vi "UHR-Fleezers Control (host) - 12.6.vi"() -> ()   [LabVIEW 2012] (continued)
          tunnel: w2733 -> [w2738]
          tunnel: [w2736] -> w2731
          tunnel: [w2735] -> w2730
          tunnel: [w2741] -> w2729
          tunnel: w2731 -> [w2741]
          tunnel: [w2740] -> w2728
          tunnel: w2730 -> [w2740]
          tunnel: w2729 -> [w2745]
          tunnel: w2728 -> [w2744]
          tunnel: [w2743] -> w2732
          frame #0 {
            n1852 = xnode "Read/Write Control"("FPGA VI Reference In"=w2739, "error in"=w2738, "Green Filter Flipper"=TRUE) -> ("FPGA VI Reference Out"=w2736:T20, "error out"=w2735:errorcluster)
          }
          frame #1 {
            n1853 = Wait (ms)(milliseconds to wait=u32 100) -> ()  [unwired: 1 out]
          }
          frame #2 {
            n1854 = xnode "Read/Write Control"("FPGA VI Reference In"=w2745, "error in"=w2744, "Green Filter Flipper"=FALSE) -> ("error out"=w2743:errorcluster)  [unwired: 1 out]
          }
        }
      }
      event "Pump 1 contents", "Pump 3 contents": Value Change {
        n1855 = event-data() -> ()  [unwired: 7 out]
        n1856 = local read "Pump 1 contents"() -> (→"Pump 1 cont disp":string)
        n1857 = local read "Pump 3 contents"() -> (→"Pump 3 cont disp":string)
      }
      event "Reset Trap Pos. FB": Value Change {
        n1858 = event-data() -> ()  [unwired: 7 out]
        n1859 = xnode "Read/Write Control"("FPGA VI Reference In"=w2751, "error in"=w2750, "Trap Pos. FB Reset"="Reset Trap Pos. FB") -> ()  [unwired: 2 out]
      }
      event "Rem fb disp offset": Value Change {
        n1860 = event-data() -> ()  [unwired: 7 out]
        n1861 = local write "Rem fb disp offset"(FALSE ("Rem fb disp offset")) -> ()
        n1862 = local read "Mean T1 Position (nm)"() -> (w2753:dbl)
        n1863 = local read "FB Trap Pos Offset"() -> (w2754:dbl)
        n1864 = Subtract(x=w2754, y=w2753) -> (x-y=w2752:dbl)
        n1865 = local write "FB Trap Pos Offset"(w2752) -> ()
      }
      event "Threshold (nm)": Value Change {
        n1866 = event-data() -> ()  [unwired: 7 out]
        n1867 = flat-sequence {
          tunnel: w2758 -> [w2766]
          tunnel: w2757 -> [w2765]
          tunnel: [w2759] -> w2756
          tunnel: w2756 -> [w2772]
          frame #0 {
            n1868 = xnode "Read/Write Control"("FPGA VI Reference In"=w2766, "error in"=w2765) -> ("FPGA VI Reference Out"=w2762:T20, "error out"=w2761:errorcluster, "FPGA TTrig Thresh"=w2763:i64)
            n1869 = local read "Threshold stored (nm)"() -> (w2771:dbl)
            n1870 = local read "Threshold (nm)"() -> (w2759:dbl)
            n1871 = local read "AOM X Cal (nm/MHz)"() -> (w2769:dbl)
            n1872 = Subtract(x=w2759, y=w2771) -> (x-y=w2770:dbl)
            n1873 = Divide(x=w2770, y=w2769) -> (x/y=w2767:dbl)
            n1874 = call "IR AOM freq to word.vi"("Frequency In (MHz)"=w2767) -> ("Frequency Word Out (double)"=w2768:dbl)
            n1875 = To Quad Integer(1:w2768) -> (0:w2764:i64)
            n1876 = Add(x=w2763, y=w2764) -> (x+y=w2760:i64)
            n1877 = xnode "Read/Write Control"("FPGA VI Reference In"=w2762, "error in"=w2761, "FPGA TTrig Thresh"=w2760) -> ()  [unwired: 2 out]
          }
          frame #1 {
            "Threshold stored (nm)" <- w2772
          }
        }
      }
      event "FB Trig Integrate": Value Change {
        n1878 = event-data() -> ()  [unwired: 7 out]
        n1879 = local read "FB Trig Integrate"() -> (w2774:u32)
        n1880 = xnode "Read/Write Control"("FPGA VI Reference In"=w2776, "error in"=w2775, "FB Trig Integrate"=w2774) -> ("error out"=w2773:errorcluster)  [unwired: 1 out]
      }
      event "11": Value Change {
        n1881 = event-data() -> ()  [unwired: 7 out]
        n1882 = local read "11"() -> (w2777:bool)
        n1883 = case shown="True" w2777 {
          frame False {
          }
          frame True {
            n1884 = local read "Messages"() -> (w2779:string)
            n1885 = call "Update messages.vi"("Message to add"="You kicked it up to 11!", "Old message string"=w2779) -> ("New message string"=w2780:string)
            n1886 = call <vilib>:"Beep.vi"() -> ()  [unwired: 12 in]
            n1887 = local write "Messages"(w2780) -> ()
          }
        }
      }
      event "Trap Pos. FB ON": Value Change {
        n1888 = event-data() -> ()  [unwired: 7 out]
        n1889 = xnode "Read/Write Control"("FPGA VI Reference In"=w2783, "error in"=w2782, "Force feedback"="Trap Pos. FB ON") -> ()  [unwired: 2 out]
      }
      event "Remove Action Offset": Value Change {
        n1890 = event-data() -> ()  [unwired: 7 out]
        n1891 = local write "Remove Action Offset"(FALSE ("Remove Action Offset")) -> ()
        n1892 = local read "Trap Pos. FB Mult Factor"() -> (w2788:i64)
        n1893 = local read "Trap Pos FB Action"() -> (w2786:i64)
        n1894 = local read "Trap Pos. FB Offset Factor"() -> (w2784:i64)
        n1895 = Multiply(x=w2788, y=w2786) -> (x*y=w2787:i64)
        n1896 = Add(x=w2787, y=w2784) -> (x+y=w2785:i64)
        n1897 = local write "Trap Pos. FB Offset Factor"(w2785) -> ()
        n1898 = xnode "Read/Write Control"("FPGA VI Reference In"=w2791, "error in"=w2790, "Trap Pos. FB Offset Factor"=w2785) -> ()  [unwired: 2 out]
      }
      event "Remove Unwinding Offset": Value Change {
        n1899 = event-data() -> ()  [unwired: 7 out]
        n1900 = local write "Remove Unwinding Offset"(FALSE ("Remove Action Offset")) -> ()
        n1901 = local read "Trap Pos. FB Mult Factor"() -> (w2803:i64)
        n1902 = local read "Trap Pos FB Action"() -> (w2801:i64)
        n1903 = local read "Trap Pos. FB Offset Factor"() -> (w2800:i64)
        n1904 = Multiply(x=w2803, y=w2801) -> (x*y=w2802:i64)
        n1905 = local read "Trap Pos. FB Mult Factor"() -> (w2799:i64)
        n1906 = Add(x=w2802, y=w2800) -> (x+y=w2793:i64)
        n1907 = Multiply(x=32768, y="factor") -> (x*y=w2796:dbl)
        n1908 = Multiply(x=w2796, y=w2799) -> (x*y=w2798:dbl)
        n1909 = Subtract(x=w2793, y=w2798) -> (x-y=w2797:dbl)
        n1910 = To Quad Integer(1:w2797) -> (0:w2792:i64)
        n1911 = xnode "Read/Write Control"("FPGA VI Reference In"=w2806, "error in"=w2805, "Trap Pos. FB Offset Factor"=w2792) -> ()  [unwired: 2 out]
        n1912 = local write "Trap Pos. FB Offset Factor"(w2792) -> ()
      }
      event "Trap Pos. FB Range", "Trap Pos. FB Gains", "Trap Pos. FB Mult Factor", "Trap Pos. FB Offset Factor", "Trap Pos FB Negate Action", "Trap Pos FB Monitor\nT1 or T2", "Differential FB?", "Negate Diff?": Value Change {
        n1913 = event-data() -> ()  [unwired: 7 out]
        n1914 = Unbundle By Name("Trap Pos. FB Gains") -> ("proportional gain (Kc)"=w2809:fxp<+/-,16,8>, "integral gain (Kc*Ts/Ti)"=w2808:fxp<+/-,16,8>, "derivative gain (Kc*Td/Ts)"=w2807:fxp<+/-,16,8>)
        n1915 = local read "Negate Diff?"() -> (w2814:bool)
        n1916 = Unbundle By Name("Trap Pos. FB Range") -> ("output high"=w2812:fxp<+/-,16,1>, "output low"=w2811:fxp<+/-,16,1>)
        n1917 = xnode "Read/Write Control"("FPGA VI Reference In"=w2822, "error in"=w2821, "FB2 output high"=w2812, "FB2 output low"=w2811, "P2"=w2809, "I2"=w2808, "D2"=w2807, "Trap Pos. FB Mult Factor"="Trap Pos. FB Mult Factor", "Trap Pos. FB Offset Factor"="Trap Pos. FB Offset Factor", "Trap Pos FB Negate Action"="Trap Pos FB Negate Action", "Trap Pos FB Monitor T1 or T2"="Trap Pos FB Monitor\nT1 or T2", "AI1 X Scale"="Trap Pos. AI1 X Pre-scale", "Negate Diff?"=w2814, "Diff FB Measurement?"="Differential FB?") -> ()  [unwired: 2 out]
      }
      event "Trap Pos FB SP", "Trap Pos FB SP 2", "Use SP 2": Value Change {
        n1918 = event-data() -> ()  [unwired: 7 out]
        n1919 = Select(t="Trap Pos FB SP 2", s="Use SP 2", f="Trap Pos FB SP") -> (s? t:f=w2823:fxp<+/-,16,1>)
        n1920 = xnode "Read/Write Control"("FPGA VI Reference In"=w2828, "error in"=w2827, "Trap Pos. FB SP"=w2823) -> ()  [unwired: 2 out]
      }
      event "Offset SP2 from SP1": Value Change {
        n1921 = event-data() -> ()  [unwired: 7 out]
        n1922 = local read "Trap Pos FB SP"() -> (w2831:fxp<+/-,16,1>)
        n1923 = Add(x=w2831, y="SP2 Offset") -> (x+y=w2829:fxp<+/-,16,1>)
        n1924 = property on="Trap Pos FB SP 2" class="DigNum (strict)"("Val(Sgnl)"=w2829) -> ()  [unwired: 2 in, 2 out]
        n1925 = local write "Offset SP2 from SP1"(FALSE ("Offset SP2 from SP1")) -> ()
      }
      event "Set Reading to\nSetpoint": Value Change {
        # "This is the actual PID input signal"
        n1926 = event-data() -> ()  [unwired: 7 out]
        n1927 = local write "Set Reading to\nSetpoint"(FALSE ("Set SP to Reading")) -> ()
        n1928 = xnode "Read/Write Control"("FPGA VI Reference In"=w2837, "error in"=w2836) -> ("FPGA VI Reference Out"=w2835:T20, "error out"=w2834:errorcluster, "Trap Pos FB Int-Norm Signal"=w2833:fxp<+/-,16,1>)
        n1929 = local read "Differential FB?"() -> (w2838:bool)
        n1930 = case shown="False" w2838 {
          tunnel: [w2843 w2850] -> w2840
          tunnel: w2833 -> [w2841 w2850]
          frame False {
            n1931 = local read "Trap Pos FB Monitor\nT1 or T2"() -> (w2846:bool)
            n1932 = local read "Trap X AI1 (DMA)"() -> (w2849:T13)
            n1933 = Unbundle By Name(w2849) -> ("Set 1"=w2848:fxp<+/-,16,1>, "Set 2"=w2847:fxp<+/-,16,1>)
            n1934 = Select(t=w2848, s=w2846, f=w2847) -> (s? t:f=w2845:fxp<+/-,16,1>)
            n1935 = Not(x="Set SP Using...") -> (.not. x?=w2842:bool)
            n1936 = Select(t=w2841, s=w2842, f=w2845) -> (s? t:f=w2843:fxp<+/-,16,1>)
          }
          frame True {
          }
        }
        n1937 = xnode "Read/Write Control"("FPGA VI Reference In"=w2835, "error in"=w2834, "Trap Pos. FB SP"=w2840) -> ()  [unwired: 2 out]
        n1938 = local write "Trap Pos FB SP"(w2840) -> ()
      }
      event "Trap Pos. FB Out Scale 2^n": Value Change {
        n1939 = event-data() -> ()  [unwired: 7 out]
        n1940 = Scale By Power Of 2(n="Trap Pos. FB Out Scale 2^n", x=ext 1.0) -> (x*2^n=w2851:ext)
        n1941 = property on="Trap Pos. FB Mult Factor" class="DigNum (strict)"("Val(Sgnl)"=w2851) -> ()  [unwired: 2 in, 2 out]
      }
      event "Trap Pos FB Int Count": Value Change {
        n1942 = event-data() -> ()  [unwired: 7 out]
        n1943 = xnode "Read/Write Control"("FPGA VI Reference In"=w2856, "error in"=w2855, "Trap Pos FB Int Count"="Trap Pos FB Int Count") -> ()  [unwired: 2 out]
      }
      event "Trap pos": Value Change {
        n1944 = event-data() -> ()  [unwired: 7 out]
        n1945 = case shown="True" "Trap pos" {
          frame False {
            n1946 = property on="Trap Delta Graph" class="WFGraph (strict)"("Visible"=TRUE) -> ()  [unwired: 2 in, 2 out]
            n1947 = property on="Saved trap pos" class="WFGraph (strict)"("Visible"=FALSE) -> ()  [unwired: 2 in, 2 out]
          }
          frame True {
            n1948 = property on="Saved trap pos" class="WFGraph (strict)"("Visible"=TRUE) -> ()  [unwired: 2 in, 2 out]
            n1949 = property on="Trap Delta Graph" class="WFGraph (strict)"("Visible"=FALSE) -> ()  [unwired: 2 in, 2 out]
          }
        }
      }
    }
    "error out 2" <- w1685
    n1950 = node-c288() -> ()  [unwired: 2 out]
  }
  n1951 = while "Duncan's play event loop" {
    stop <- w2863 stop-if-true
    n1952 = Create User Event(user event datatype=TRUE ("Boolean")) -> (user event=w2864:refnum<user-event>)  [unwired: 1 in, 1 out]
    n1953 = Create User Event(user event datatype=TRUE ("Boolean")) -> (user event=w2871:refnum<user-event>)  [unwired: 1 in, 1 out]
    n1954 = global write "Global for fluorescence simulation mean (30 samples), (power series).vi" "Red Signal"(w2864) -> ()
    n1955 = global write "Global for fluorescence simulation mean (30 samples), (power series).vi" "Green Signal"(w2871) -> ()
    n1956 = register-events(w2871, w2864) -> (reference out=w2870:refnum<event-registration>)  [unwired: 2 in, 1 out]
    n1957 = event shown="[1] \"Get Fluorophore\": Value Change" {
      selector: w2870 -> [_ _ _ _]
      dyn-events: _ -> [_ _ _ _]
      timeout: 100 -> [_ _ _ _]
      event Timeout {
        n1958 = event-data() -> ()  [unwired: 1 in, 2 out]
      }
      event "Get Fluorophore": Value Change {
        n1959 = event-data() -> ("OldVal"=w2873:bool)  [unwired: 1 in, 4 out]
        n1960 = case shown="True" w2873 {
          selector: w2873 -> [_ w2874]
          frame False {
          }
          frame True {
            n1961 = property on="Move to Position 3" class="Bool"("Val(Sgnl)"=w2874) -> ()  [unwired: 2 in, 2 out]
            n1962 = case shown="1" "Numeric" {
              frame 0, Default {
              }
              frame 1 {
                n1963 = property on="Green Laser ON" class="Bool (strict)"("Val(Sgnl)"=TRUE ("Value (Signaling)")) -> ()  [unwired: 2 in, 2 out]
              }
              frame 2 {
                n1964 = property on="Red Laser ON" class="Bool (strict)"("Val(Sgnl)"=TRUE) -> ()  [unwired: 2 in, 2 out]
              }
            }
          }
        }
      }
      event User Event {
        n1965 = event-data() -> ("Boolean"=w2878:bool)  [unwired: 1 in, 3 out]
        "Green Fluorophore" <- w2878
        n1966 = property on="Get Fluorophore" class="Bool (strict)"("Val(Sgnl)"=w2878) -> ()  [unwired: 2 in, 2 out]
      }
      event User Event {
        n1967 = event-data() -> ("Boolean"=w2879:bool)  [unwired: 1 in, 3 out]
        "Red Fluorophore" <- w2879
        n1968 = property on="Get Fluorophore" class="Bool (strict)"("Val(Sgnl)"=w2879) -> ()  [unwired: 2 in, 2 out]
      }
    }
    n1969 = property on="Get Fluorophore" class="Bool (strict)"("Val(Sgnl)"="Get Fluorophore") -> ()  [unwired: 2 in, 2 out]
    n1970 = Wait (ms)(milliseconds to wait=u32 100) -> ()  [unwired: 1 out]
    n1971 = local read "Stop All"() -> (w2862:bool)
    n1972 = Or(x=w2862, y="stop") -> (x .or. y?=w2863:bool)
  }
  n1973 = timed-loop "Mouse control: trap position (AOM deflection), set confocal spot from image" {
    tunnel: [w2881] -> w206
    tunnel: w16 -> [w2880]
    timing: w128 -> [_]
    timing-out: [_] -> w127
    stop <- w2881 stop-if-true
    n1974 = node-c288() -> ()  [unwired: 2 out]
    n1975 = event shown="[0] \"Pane\": Mouse Down" {
      selector: _ -> [_ _]
      dyn-events: _ -> [_ _]
      timeout: _ -> [_ _]
      tunnel: w2880 -> [w2884 _]
      event Mouse Down {
        n1976 = event-data() -> ("Time"=w2886:u32, "Coords"=w2885:T7, "Button"=w2887:u16)  [unwired: 6 out]
        n1977 = case shown="3" w2887 {
          tunnel: w2886 -> [_ _ w2993]
          tunnel: w2885 -> [_ w2924 w2991]
          tunnel: w2884 -> [_ _ w2989]
          frame 0, Default {
          }
          frame 1 {
            n1978 = property on="APD 2" class="ImageControl"() -> ("Displayed Image Position"=w2894:cluster{"Left":i32, "Top":i32})  [unwired: 2 in, 2 out]
            n1979 = property on="APD 1" class="ImageControl"() -> ("Displayed Image Position"=w2923:cluster{"Left":i32, "Top":i32})  [unwired: 2 in, 2 out]
            n1980 = property on="Detection Laser X" class="ImageControl"() -> ("Displayed Image Position"=w2920:cluster{"Left":i32, "Top":i32})  [unwired: 2 in, 2 out]
            n1981 = property on="Detection Laser Y" class="ImageControl"() -> ("Displayed Image Position"=w2919:cluster{"Left":i32, "Top":i32})  [unwired: 2 in, 2 out]
            n1982 = property on="APD 2" class="ImageControl"() -> ("Displayed Image Size"=w2893:cluster{"Width":u32, "Height":u32})  [unwired: 2 in, 2 out]
            n1983 = property on="APD 1" class="ImageControl"() -> ("Displayed Image Size"=w2921:cluster{"Width":u32, "Height":u32})  [unwired: 2 in, 2 out]
            n1984 = property on="Detection Laser X" class="ImageControl"() -> ("Displayed Image Size"=w2922:cluster{"Width":u32, "Height":u32})  [unwired: 2 in, 2 out]
            n1985 = property on="Detection Laser Y" class="ImageControl"() -> ("Displayed Image Size"=w2918:cluster{"Width":u32, "Height":u32})  [unwired: 2 in, 2 out]
            n1986 = Unbundle By Name(w2893) -> ("Width"=w2890:u32, "Height"=w2889:u32)
            n1987 = Unbundle By Name(w2894) -> ("Left"=w2892:i32, "Top"=w2891:i32)
            n1988 = Unbundle By Name(w2921) -> ("Width"=w2915:u32, "Height"=w2914:u32)
            n1989 = Unbundle By Name(w2922) -> ("Width"=w2911:u32, "Height"=w2910:u32)
            n1990 = Unbundle By Name(w2918) -> ("Width"=w2907:u32, "Height"=w2906:u32)
            n1991 = Unbundle By Name(w2923) -> ("Left"=w2917:i32, "Top"=w2916:i32)
            n1992 = Unbundle By Name(w2920) -> ("Left"=w2913:i32, "Top"=w2912:i32)
            n1993 = Unbundle By Name(w2919) -> ("Left"=w2909:i32, "Top"=w2908:i32)
            n1994 = Bundle("Left"=w2892, "Top"=w2891, "Width"=w2890, "Height"=w2889) -> (w2888:T33)  [unwired: 1 in]
            n1995 = Bundle("Left"=w2917, "Top"=w2916, "Width"=w2915, "Height"=w2914) -> (w2905:T33)  [unwired: 1 in]
            n1996 = Bundle("Left"=w2913, "Top"=w2912, "Width"=w2911, "Height"=w2910) -> (w2904:T33)  [unwired: 1 in]
            n1997 = Bundle("Left"=w2909, "Top"=w2908, "Width"=w2907, "Height"=w2906) -> (w2903:T33)  [unwired: 1 in]
            n1998 = Build Cluster Array(w2888, w2905, w2904, w2903) -> (w2902:T34)
            n1999 = for {
              tunnel: w2924 -> [w2935]
              tunnel: w2902 -> [w2936] mode=indexing
              shift-right: [w2933] -> w2900
              shift-left: TRUE -> [w2934]
              shift-right: [w2932] -> w2898
              shift-left: _ -> [w2928]
              shift-right: [w2931] -> w2897
              shift-left: _ -> [w2927]
              shift-right: [w2930] -> w2896
              shift-left: _ -> [w2926]
              shift-right: [w2929] -> w2895
              shift-left: _ -> [w2925]
              n2000 = case shown="True" w2934 {
                selector: w2934 -> [w2941 _]
                tunnel: w2936 -> [_ w2950]
                tunnel: w2935 -> [_ w2948]
                tunnel: [w2941 w2946] -> w2933
                tunnel: [w2940 w2945] -> w2932
                tunnel: [w2939 w2944] -> w2931
                tunnel: [w2938 w2943] -> w2930
                tunnel: [w2937 w2942] -> w2929
                tunnel: w2928 -> [w2940 _]
                tunnel: w2927 -> [w2939 _]
                tunnel: w2926 -> [w2938 _]
                tunnel: w2925 -> [w2937 _]
                frame False {
                }
                frame True {
                  n2001 = Unbundle(w2950) -> (w2949:T33)
                  n2002 = call "isclickinwindow.vi"("Image Param"=w2949, "Point32"=w2948) -> ("4 Y"=w2942:i32, "3 Height"=w2943:i32, "2 X"=w2944:i32, "1 Width"=w2945:i32, "In image?"=w2947:bool)  [unwired: 1 in]
                  n2003 = Not(x=w2947) -> (.not. x?=w2946:bool)
                }
              }
            }
            n2004 = Not(x=w2900) -> (.not. x?=w2899:bool)
            n2005 = case shown="True" w2899 {
              tunnel: w2897 -> [_ w2964]
              tunnel: w2895 -> [_ w2963]
              tunnel: w2898 -> [_ w2962]
              tunnel: w2896 -> [_ w2961]
              frame False {
              }
              frame True {
                w2951 = FALSE ("Get Point")
                n2006 = local read "Scan lines (y)"() -> (w2966:u64)
                n2007 = disable-structure shown="Disabled" {
                  frame Disabled {
                  }
                  frame Enabled {
                  }
                }
                n2008 = local read "Actual MCL Inc (V)"() -> (w2960:dbl)
                n2009 = local read "Scan steps (MCL)"() -> (w2965:u64)
                n2010 = Divide "Y Pix/step"(x=w2961, y=w2966) -> (x/y=w2973:dbl)
                n2011 = Divide "Y V/pix"(x=w2960, y=w2973) -> (x/y=w2972:dbl)
                n2012 = Divide "Y half step offset"(x=w2960, y=2.0) -> (x/y=w2974:dbl)
                n2013 = Divide "X pix/step"(x=w2962, y=w2965) -> (x/y=w2971:dbl)
                n2014 = Negate(x=w2974) -> (-x=w2975:dbl)
                n2015 = local read "Initial Y"() -> (w2981:dbl)
                n2016 = Multiply(x=w2963, y=w2972) -> (x*y=w2982:dbl)
                n2017 = Divide "X half step offset"(x=w2960, y=2.0) -> (x/y=w2968:dbl)
                n2018 = Divide "X V/pix"(x=w2960, y=w2971) -> (x/y=w2970:dbl)
                n2019 = Multiply(x=w2960, y=w2965) -> (x*y=w2977:dbl)
                n2020 = Compound Arithmetic op=ADD(w2975, w2982, w2981) -> (w2952:dbl)
                "Pointer Y (V)" <- w2952
                n2021 = Multiply(x=w2970, y=w2964) -> (x*y=w2979:dbl)
                n2022 = Negate(x=w2968) -> (-x=w2967:dbl)
                n2023 = local read "Initial X"() -> (w2980:dbl)
                n2024 = Negate(x=w2979) -> (-x=w2978:dbl)
                n2025 = Compound Arithmetic op=ADD(w2967, w2977, w2980, w2978) -> (w2953:dbl)
                "Pointer X (V)" <- w2953
                n2026 = case shown="True" "Set High F Confocal Spot (X-Y)" {
                  tunnel: w2953 -> [_ w2983]
                  tunnel: w2952 -> [_ w2984]
                  frame False {
                  }
                  frame True {
                    "Confocal Y 2 (V)" <- w2984
                    "Confocal X 2 (V)" <- w2983
                  }
                }
                n2027 = Or(x="Set X Only", y="Set Confocal Spot (X-Y)") -> (x .or. y?=w2956:bool)
                n2028 = Or(x="Set Confocal Spot (X-Y)", y="Set Y Only") -> (x .or. y?=w2955:bool)
                n2029 = case shown="True" w2956 {
                  tunnel: w2953 -> [_ w2985]
                  frame False {
                  }
                  frame True {
                    n2030 = property on="AO2" class="Slide (strict)"("Val(Sgnl)"=w2985) -> ()  [unwired: 2 in, 2 out]
                    "Confocal X 1 (V)" <- w2985
                  }
                }
                n2031 = case shown="True" w2955 {
                  tunnel: w2952 -> [_ w2986]
                  frame False {
                  }
                  frame True {
                    n2032 = property on="AO1" class="Slide (strict)"("Val(Sgnl)"=w2986) -> ()  [unwired: 2 in, 2 out]
                    "Confocal Y 1 (V)" <- w2986
                  }
                }
                n2033 = local write "Set High F Confocal Spot (X-Y)"(w2951) -> ()
                n2034 = local write "Set Confocal Spot (X-Y)"(w2951) -> ()
                n2035 = local write "Set X Only"(w2951) -> ()
                n2036 = local write "Set Y Only"(w2951) -> ()
              }
            }
          }
          frame 3 {
            n2037 = local read "BD 2 Frequency 1 (MHz)"() -> (w2987:dbl)
            n2038 = local read "BD 1 Frequency 1 (MHz)"() -> (w2988:dbl)
            n2039 = local write "Manipulating Trap"(TRUE ("Manipulating Trap")) -> ()
            n2040 = local write "Coords"(T7 {"Horizontal"=0, "Vertical"=0} ("Coords")) -> ()
            n2041 = while {
              tunnel: w2993 -> [w2998]
              tunnel: w2991 -> [w2997]
              tunnel: w2989 -> [w2996]
              tunnel: w2988 -> [w2995]
              tunnel: w2987 -> [w2994]
              stop <- w2999 stop-if-true
              n2042 = event shown="[0] \"Pane\": Mouse Move" {
                selector: _ -> [_ _]
                dyn-events: _ -> [_ _]
                timeout: _ -> [_ _]
                tunnel: ["Force Manip Abort" w3063] -> w2999
                tunnel: w2998 -> [w3006 _]
                tunnel: w2997 -> [w3004 _]
                tunnel: w2996 -> [w3003 _]
                tunnel: w2995 -> [w3002 _]
                tunnel: w2994 -> [w3001 _]
                event Mouse Move {
                  n2043 = event-data() -> ("Time"=w3007:u32, "Coords"=w3008:T7)  [unwired: 3 out]
                  n2044 = Less?(x=w3007, y=w3006) -> (x < y?=w3005:bool)
                  n2045 = case "Makes sure old motion events prior to mouse click aren't used" shown="False" w3005 {
                    tunnel: w3008 -> [w3050 _]
                    tunnel: w3004 -> [w3051 _]
                    tunnel: w3003 -> [w3028 _]
                    tunnel: w3002 -> [w3024 _]
                    tunnel: w3001 -> [w3023 _]
                    frame False {
                      n2046 = Subtract(x=w3050, y=w3051) -> (x-y=w3049:T7)
                      "Coords" <- w3049
                      n2047 = local read "Y RF Frequency Limits (MHz)"() -> (w3009:T16)
                      n2048 = To Double Precision Float(number=w3049) -> (double precision float=w3048:cluster{"Horizontal":dbl, "Vertical":dbl})
                      n2049 = Multiply(x=cluster{"Horizontal":dbl, "Vertical":dbl} {"Horizontal"=-1.0, "Vertical"=1.0}, y="Manipulation Scaling") -> (x*y=w3044:cluster{"Horizontal":dbl, "Vertical":dbl})
                      n2050 = local read "X RF Frequency Limits (MHz)"() -> (w3010:T16)
                      n2051 = Multiply(x=w3048, y=w3044) -> (x*y=w3046:cluster{"Horizontal":dbl, "Vertical":dbl})
                      n2052 = Unbundle By Name(w3046) -> ("Horizontal"=w3041:dbl, "Vertical"=w3045:dbl)
                      n2053 = Unbundle By Name(w3009) -> ("Maximum"=w3012:dbl, "Minimum"=w3011:dbl)
                      n2054 = Boolean To (0,1)(Boolean="Manip. X?") -> (0, 1=w3039:i16)
                      n2055 = Boolean To (0,1)(Boolean="Manip. Y?") -> (0, 1=w3036:i16)
                      n2056 = local read "BD 1 Frequency 2 (MHz)"() -> (w3026:dbl)
                      n2057 = Multiply(x=w3045, y=w3036) -> (x*y=w3038:dbl)
                      n2058 = Multiply(x=w3039, y=w3041) -> (x*y=w3042:dbl)
                      n2059 = local read "BD 2 Frequency 2 (MHz)"() -> (w3025:dbl)
                      n2060 = Unbundle By Name(w3010) -> ("Maximum"=w3014:dbl, "Minimum"=w3013:dbl)
                      n2061 = Add(x=w3023, y=w3038) -> (x+y=w3016:dbl)
                      n2062 = Add(x=w3024, y=w3042) -> (x+y=w3018:dbl)
                      n2063 = In Range and Coerce(upper limit=w3014, x=w3018, lower limit=w3013) -> (coerced(x)=w3017:dbl)  [unwired: 1 out]
                      n2064 = In Range and Coerce(upper limit=w3012, x=w3016, lower limit=w3011) -> (coerced(x)=w3015:dbl)  [unwired: 1 out]
                      n2065 = Subtract(x=w3017, y=w3026) -> (x-y=w3035:dbl)
                      n2066 = Subtract(x=w3015, y=w3025) -> (x-y=w3034:dbl)
                      n2067 = Square(x=w3035) -> (x^2=w3033:dbl)
                      n2068 = Square(x=w3034) -> (x^2=w3032:dbl)
                      n2069 = Add(x=w3033, y=w3032) -> (x+y=w3031:dbl)
                      n2070 = Square Root(x=w3031) -> (sqrt(x)=w3027:dbl)
                      n2071 = In Range and Coerce(upper limit="Limit Max (MHz)", x=w3027, lower limit="Limit Min (MHz)") -> (In Range?=w3020:bool)  [unwired: 1 out]
                      n2072 = Not(x="Limits Enable") -> (.not. x?=w3019:bool)
                      n2073 = Or(x=w3020, y=w3019) -> (x .or. y?=w3021:bool)
                      n2074 = case shown="True" w3021 {
                        tunnel: w3028 -> [_ w3061]
                        tunnel: w3027 -> [_ w3052]
                        tunnel: w3017 -> [_ w3059]
                        tunnel: w3026 -> [_ w3058]
                        tunnel: w3015 -> [_ w3057]
                        tunnel: w3025 -> [_ w3056]
                        tunnel: w3010 -> [_ w3054]
                        tunnel: w3009 -> [_ w3053]
                        frame False {
                        }
                        frame True {
                          n2075 = local read "BD 1 Frequency 3 (MHz)"() -> (w3060:dbl)
                          n2076 = local read "BD 2 Frequency 3 (MHz)"() -> (w3055:dbl)
                          n2077 = local write "Trap Delta (MHz)"(w3052) -> ()
                          n2078 = call "set RF board frequency - interlace.vi"("Board 2 Frequency Limits"=w3053, "Board 1 Frequency Limits"=w3054, "FPGA VI Reference In"=w3061, "Board 2 Frequency 3 (MHz)"=w3055, "Board 1 Frequency 3 (MHz)"=w3060, "Board 2 Frequency 2 (MHz)"=w3056, "Board 2 Frequency 1 (MHz)"=w3057, "Board 1 Frequency 2 (MHz)"=w3058, "Board 1 Frequency 1  (MHz)"=w3059) -> ()  [unwired: 1 in, 2 out]
                          n2079 = local write "BD 2 Frequency 1 (MHz)"(w3057) -> ()
                          n2080 = local write "BD 1 Frequency 1 (MHz)"(w3059) -> ()
                        }
                      }
                    }
                    frame True {
                    }
                  }
                }
                event Mouse Up {
                  n2081 = event-data() -> ("Button"=w3062:u16)  [unwired: 8 out]
                  n2082 = case shown="3" w3062 {
                    tunnel: [FALSE TRUE] -> w3063
                    frame 0, Default {
                    }
                    frame 3 {
                      n2083 = local read "Trap Delta (MHz)"() -> (w3065:dbl)
                      n2084 = property on="Initial delta (MHz)" class="DigNum (strict)"("Val(Sgnl)"=w3065) -> ()  [unwired: 2 in, 2 out]
                      n2085 = local write "Manipulating Trap"(FALSE ("Manipulating Trap")) -> ()
                    }
                  }
                }
              }
            }
          }
        }
      }
      event Mouse Move {
        n2086 = event-data() -> ()  [unwired: 6 out]
      }
    }
    n2087 = local read "Stop All"() -> (w2881:bool)
    n2088 = node-c288() -> ()  [unwired: 2 out]
  }
  n2089 = timed-loop "Main data acquisition loop (get data, process data for display, and save data to disk)" {
    tunnel: w15 -> [w3377]
    tunnel: w87 -> [w3376]
    tunnel: [w3406] -> w291
    tunnel: [w3401] -> w289
    timing: w199 -> [_]
    timing-out: [_] -> w198
    tunnel: w104 -> [w3230]
    stop <- "Stop All" stop-if-true
    w3147 = "Initialize"
    # "Fluorescence data into FIFO for external control vi's\n(e.g., fluorescence triggering) - Duncan Nall"
    n2090 = node-c288() -> ()  [unwired: 2 out]
    n2091 = First Call?() -> (First Call?: T/F=w3182:bool)
    n2092 = Or(x="Reset", y=w3182) -> (x .or. y?=w3183:bool)
    n2093 = local read "Flushing P1"() -> (w3102:bool)
    n2094 = case "Reset data stream (manual reset or at begining of some rastering and imaging)" shown="True" w3183 {
      tunnel: w3377 -> [w4447 w4455]
      tunnel: w3376 -> [w4446 w4454]
      tunnel: [w4447 w4449] -> w3372
      tunnel: [w4446 w4448] -> w3371
      frame False {
      }
      frame True {
        w4452 = TRUE ("AI to FIFO")
        n2095 = local write "Overflow (data lost)"(FALSE ("Overflow (data lost)")) -> ()
        n2096 = call "reset FPGA DMA.vi"("error in"=w4454, "FPGA VI Reference In"=w4455) -> ("error out"=w4450:errorcluster, "FPGA VI Reference Out"=w4451:T20)
        n2097 = xnode "Read/Write Control"("FPGA VI Reference In"=w4451, "error in"=w4450, "AI to FIFO"=w4452, "APD to FIFO"=w4452) -> ("FPGA VI Reference Out"=w4449:T20, "error out"=w4448:errorcluster)
      }
    }
    n2098 = case shown="True" w3102 {
      frame False {
      }
      frame True {
        n2099 = local read "Flush rate (uL/m) P1"() -> (w3436:dbl)
        n2100 = local read "HP1 Flush Time (s)"() -> (w3445:dbl)
        n2101 = local read "DMA Update Period (s)"() -> (w3439:dbl)
        n2102 = Divide(x=w3436, y=60.0) -> (x/y=w3437:dbl)
        n2103 = Divide(x=w3445, y=w3439) -> (x/y=w3434:dbl)
        n2104 = feedback #1(0) -> (w3443:i32)
        n2105 = Increment(x=w3443) -> (x+1=w3433:i32)
        n2106 = Greater?(x=w3433, y=w3434) -> (0:w3442:bool)
        n2107 = Compound Arithmetic op=MULTIPLY(w3439, w3433, w3437) -> (→"P1 Flush Volume (uL)":dbl)
        n2108 = Divide(x=w3433, y=w3434) -> (x/y=→"P1 Flushing Bar":dbl)
        n2109 = case shown="True" w3442 {
          tunnel: w3433 -> [w3446 _]
          tunnel: [w3446 0] -> w3441
          frame False {
          }
          frame True {
            w3447 = FALSE ("Flushing P1")
            n2110 = local write "Inject Pump 1"(w3447) -> ()
            n2111 = local write "Flushing P1"(w3447) -> ()
            n2112 = property on="Clear Volume P1" class="Bool (strict)"("Val(Sgnl)"=TRUE ("Value (Signaling)")) -> ()  [unwired: 2 in, 2 out]
          }
        }
        n2113 = feedback-in #1(w3441) -> ()
      }
    }
    n2114 = Or(x="Start AOD Scan", y="Trap Raster Scan") -> (x .or. y?=w3328:bool)
    n2115 = case "Start AOM raster scan" shown="True" w3328 {
      tunnel: w3372 -> [w4297 w4307]
      tunnel: w3371 -> [w4296 w4306]
      tunnel: [w4297 w4300] -> w3370
      tunnel: [w4296 w4299] -> w3369
      frame False {
      }
      frame True {
        n2116 = case shown="True" "Restart DMA? (AOD)" {
          tunnel: [w4345 w4347] -> w4301
          tunnel: [w4344 w4346] -> w4302
          tunnel: w4307 -> [w4345 w4349]
          tunnel: w4306 -> [w4344 w4348]
          frame False {
          }
          frame True {
            n2117 = local write "Overflow (data lost)"(FALSE ("Overflow (data lost)")) -> ()
            n2118 = call "reset FPGA DMA.vi"("error in"=w4348, "FPGA VI Reference In"=w4349) -> ("error out"=w4346:errorcluster, "FPGA VI Reference Out"=w4347:T20)
          }
        }
        n2119 = local write "Trap Raster Scan"(FALSE ("Trap Raster Scan")) -> ()
        n2120 = case shown="True" "Move MCL Also?" {
          tunnel: w4302 -> [w4310 w4339]
          tunnel: w4301 -> [w4311 w4340]
          tunnel: [w4309 w4343] -> w4300
          tunnel: [w4308 w4342] -> w4299
          frame False {
            w4312 = TRUE ("AI to FIFO")
            n2121 = xnode "Read/Write Control"("FPGA VI Reference In"=w4311, "error in"=w4310, "AI to FIFO"=w4312, "APD to FIFO"=w4312, "Start scan"=w4312) -> ("FPGA VI Reference Out"=w4309:T20, "error out"=w4308:errorcluster)
          }
          frame True {
            w4336 = FALSE ("1D or 2D Scan?")
            w4341 = TRUE ("AI to FIFO")
            # "Count for MCL loop"
            # "N total cycles"
            # "N steps"
            # "V_int"
            n2122 = local read "Scan Range (nm)"() -> (w4318:dbl)
            n2123 = local read "Number of F/B Scans (AOD)"() -> (w4335:u16)
            n2124 = Sign(1:w4318) -> (0:w4317:dbl)
            n2125 = Compound Arithmetic op=MULTIPLY(w4318, "MCL Step Position Ratio", "MCL/AOM Scale Tweak") -> (w4322:dbl)
            n2126 = Negate(x=w4317) -> (-x=w4314:dbl)
            n2127 = Multiply(x=w4314, y="MCL Step Increment (V_int)") -> (x*y=w4316:dbl)
            n2128 = Divide(x=w4322, y="MCL X Cal (nm/V)") -> (x/y=w4328:dbl)
            n2129 = Multiply(x=32767.0 ("y"), y=w4328) -> (x*y=w4334:dbl)
            n2130 = local read "Total Counts (ticks)"() -> (w4319:u16)
            n2131 = local read "Cycles/step (AOD)"() -> (w4330:u64)
            n2132 = local read "Scan steps (AOD)"() -> (w4331:u64)
            n2133 = Divide(x=w4334, y=10.0) -> (x/y=w4327:dbl)
            n2134 = Divide(x=w4327, y="MCL Step Increment (V_int)") -> (x/y=w4325:dbl)
            n2135 = Absolute Value(x=w4325) -> (abs(x)=w4313:dbl)
            n2136 = Compound Arithmetic op=MULTIPLY(w4331, w4330, w4319) -> (w4326:u64)
            n2137 = local write "wait to reset values"(w4341) -> ()
            n2138 = local write "MCL Scanning"(w4341) -> ()
            n2139 = Divide(x=w4326, y=w4313) -> (x/y=w4323:dbl)
            "MCL Count" <- w4323
            n2140 = xnode "Read/Write Control"("FPGA VI Reference In"=w4340, "error in"=w4339, "Scan steps (MCL)"=w4313, "Number of scans (MCL)"=w4335, "Cycles per step (MCL)"=u64 1, "Scan freq.  increment (MCL)"=w4316, "1D or 2D Scan?"=w4336, "MCL Scan Axis"=w4336, "Cont. Scan (MCL)"=w4336, "MCL count"=w4323) -> ("FPGA VI Reference Out"=w4338:T20, "error out"=w4337:errorcluster)
            n2141 = xnode "Read/Write Control"("FPGA VI Reference In"=w4338, "error in"=w4337, "AI to FIFO"=w4341, "APD to FIFO"=w4341, "Start scan"=w4341, "Start scan (MCL)"=w4341) -> ("FPGA VI Reference Out"=w4343:T20, "error out"=w4342:errorcluster)
          }
        }
        "Raster Scanning..." <- TRUE ("Scanning...")
      }
    }
    n2142 = local read "Flushing P3"() -> (w3103:bool)
    n2143 = case "Keep track of when Harvard Pump 3 is done flushing" shown="True" w3103 {
      frame False {
      }
      frame True {
        n2144 = local read "Flush rate (uL/m) P3"() -> (w3453:dbl)
        n2145 = local read "DMA Update Period (s)"() -> (w3455:dbl)
        n2146 = local read "HP3 Flush Time (s)"() -> (w3462:dbl)
        n2147 = Divide(x=w3453, y=60.0) -> (x/y=w3451:dbl)
        n2148 = feedback #2(0) -> (w3460:i32)
        n2149 = Increment(x=w3460) -> (x+1=w3454:i32)
        n2150 = Divide(x=w3462, y=w3455) -> (x/y=w3456:dbl)
        n2151 = Greater?(x=w3454, y=w3456) -> (0:w3459:bool)
        n2152 = Compound Arithmetic op=MULTIPLY(w3455, w3454, w3451) -> (→"P3 Flush Volume (uL)":dbl)
        n2153 = case shown="True" w3459 {
          tunnel: w3454 -> [w3463 _]
          tunnel: [w3463 0] -> w3458
          frame False {
          }
          frame True {
            w3464 = FALSE ("Flushing P3")
            n2154 = local write "Inject Pump 3"(w3464) -> ()
            n2155 = local write "Flushing P3"(w3464) -> ()
            n2156 = property on="Clear Volume P3" class="Bool (strict)"("Val(Sgnl)"=TRUE ("Value (Signaling)")) -> ()  [unwired: 2 in, 2 out]
          }
        }
        n2157 = feedback-in #2(w3458) -> ()
        n2158 = Divide(x=w3454, y=w3456) -> (x/y=→"P3 Flushing Bar":dbl)
      }
    }
    n2159 = And(x="Save scans", y=w3328) -> (x .and. y?=w3368:bool)
    n2160 = Compound Arithmetic op=OR("Start MCL Scan", "Confocal Image", "Confocal Linescan") -> (w3326:bool)
    n2161 = And(x="Save Data (MCL)", y=w3326) -> (x .and. y?=w3367:bool)
    n2162 = case "Start MCL raster scan" shown="True" w3326 {
      tunnel: w3370 -> [w3909 w3925]
      tunnel: w3369 -> [w3908 w3924]
      tunnel: [w3909 w3920] -> w3229
      tunnel: [w3908 w3919] -> w3228
      tunnel: [FALSE w3918] -> w3353
      tunnel: "Start MCL Scan" -> [_ w3913]
      tunnel: "Confocal Image" -> [_ w3912]
      tunnel: "Confocal Linescan" -> [_ _]
      frame False {
      }
      frame True {
        w3918 = TRUE
        n2163 = case shown="True" "Restart DMA? (MCL)" {
          tunnel: [w3970 w3972] -> w3923
          tunnel: [w3969 w3971] -> w3922
          tunnel: w3925 -> [w3970 w3975]
          tunnel: w3924 -> [w3969 w3974]
          frame False {
          }
          frame True {
            n2164 = call "reset FPGA DMA.vi"("error in"=w3974, "FPGA VI Reference In"=w3975) -> ("error out"=w3971:errorcluster, "FPGA VI Reference Out"=w3972:T20)
            n2165 = local write "Overflow (data lost)"(FALSE ("Overflow (data lost)")) -> ()
          }
        }
        n2166 = case shown="False" w3913 {
          selector: w3913 -> [_ w3929]
          tunnel: w3912 -> [w3928 _]
          tunnel: [w3928 w3929] -> w3911
          frame False {
            n2167 = property on="2D or 1D Scan" class="Bool (strict)"("Val(Sgnl)"=w3928) -> ()  [unwired: 2 in, 2 out]
            n2168 = property on="Confocal Image" class="Bool (strict)"("Value"=FALSE ("Start Confocal Map")) -> ()  [unwired: 2 in, 2 out]
          }
          frame True {
          }
        }
        n2169 = local write "MCL Scanning"(w3918) -> ()
        n2170 = local read "AO1"() -> (w3915:dbl)
        n2171 = local read "AO2"() -> (w3914:dbl)
        n2172 = case shown="True" "Center Scan" {
          tunnel: w3923 -> [w3936 w3968]
          tunnel: w3922 -> [w3935 w3967]
          tunnel: [w3934 w3966] -> w3920
          tunnel: [w3933 w3965] -> w3919
          tunnel: [w3931 w3952] -> w3917
          tunnel: [w3930 w3951] -> w3916
          tunnel: w3915 -> [w3931 w3957]
          tunnel: w3914 -> [w3930 w3960]
          tunnel: w3911 -> [_ _]
          frame False {
            w3932 = TRUE ("AI to FIFO")
            n2173 = xnode "Read/Write Control"("FPGA VI Reference In"=w3936, "error in"=w3935, "AI to FIFO"=w3932, "APD to FIFO"=w3932, "Start scan (MCL)"=w3932) -> ("FPGA VI Reference Out"=w3934:T20, "error out"=w3933:errorcluster)
          }
          frame True {
            w3964 = TRUE ("AI to FIFO")
            n2174 = local read "Scan steps (MCL)"() -> (w3943:u64)
            n2175 = local read "Scan lines (y)"() -> (w3939:u64)
            n2176 = local read "Fast Scan Dir"() -> (w3950:bool)
            n2177 = local read "Actual MCL Inc (V)"() -> (w3940:dbl)
            n2178 = Decrement(x=w3939) -> (x-1=w3938:u64)
            n2179 = Decrement(x=w3943) -> (x-1=w3942:u64)
            n2180 = Multiply(x=w3940, y=w3938) -> (x*y=w3937:dbl)
            n2181 = Divide(x=w3937, y=2.0) -> (x/y=w3947:dbl)
            n2182 = Multiply(x=w3940, y=w3942) -> (x*y=w3941:dbl)
            n2183 = Divide(x=w3941, y=2.0) -> (x/y=w3946:dbl)
            n2184 = Select(t=w3946, s=w3950, f=w3947) -> (s? t:f=w3945:dbl)
            n2185 = Select(t=w3947, s=w3950, f=w3946) -> (s? t:f=w3949:dbl)
            n2186 = Subtract(x=w3957, y=w3949) -> (x-y=w3948:dbl)
            n2187 = Subtract(x=w3960, y=w3945) -> (x-y=w3944:dbl)
            n2188 = local read "2D or 1D Scan"() -> (w3962:bool)
            n2189 = Not(x=w3950) -> (.not. x?=w3956:bool)
            n2190 = Not(x=w3962) -> (.not. x?=w3958:bool)
            n2191 = And(x=w3950, y=w3958) -> (x .and. y?=w3959:bool)
            n2192 = And(x=w3958, y=w3956) -> (x .and. y?=w3961:bool)
            n2193 = Select(t=w3960, s=w3961, f=w3944) -> (s? t:f=w3951:dbl)
            n2194 = Select(t=w3957, s=w3959, f=w3948) -> (s? t:f=w3952:dbl)
            n2195 = call "Volt to I16.vi"("Voltage In"=w3952) -> ("I16 Voltage Out"=w3955:i16)
            n2196 = call "Volt to I16.vi"("Voltage In"=w3951) -> ("I16 Voltage Out"=w3954:i16)
            n2197 = xnode "Read/Write Control"("FPGA VI Reference In"=w3968, "error in"=w3967, "AI to FIFO"=w3964, "APD to FIFO"=w3964, "Start scan (MCL)"=w3964, "AO1"=w3955, "AO2"=w3954) -> ("FPGA VI Reference Out"=w3966:T20, "error out"=w3965:errorcluster)
          }
        }
        "Initial Y" <- w3917
        "Initial X" <- w3916
        n2198 = local write "Tab Control 6"(T3."Imaging" ("Tab Control 6")) -> ()
        "wait to reset values" <- w3918
      }
    }
    n2199 = local read "APD Elements/DMA read"() -> (w3070:u32)
    n2200 = local read "Trap AI Elements/DMA read"() -> (w3291:u32)
    n2201 = xnode "Get APD Data"("FPGA VI Reference In"=w3229, "error in"=w3228, "Number of Elements"=w3070, "Timeout (ms)"=-1) -> ("Data"=w3260:u32[], "Elements Remaining"=→"APD FIFO Elements Remaining":u32)  [unwired: 2 out]
    n2202 = local read "Trap Pos Elements/DMA read"() -> (w3225:u32)
    n2203 = xnode "Invoke Method"("FPGA VI Reference In"=w3229, "error in"=w3228, "Number of Elements"=w3225, "Timeout (ms)"=-1) -> ("Data"=w3189:u16[], "Elements Remaining"=→"Trap Pos FIFO El Remaining":u32)  [unwired: 2 out]
    n2204 = xnode "Get Trap Data"("FPGA VI Reference In"=w3229, "error in"=w3228, "Number of Elements"=w3291, "Timeout (ms)"=-1 ("Timeout")) -> ("FPGA VI Reference Out"=w3124:T20, "error out"=w3123:errorcluster, "Data"=w3190:i16[], "Elements Remaining"=w3414:u32)
    "FIFO El. Rem." <- w3414
    n2205 = local read "DMA Update Period (s)"() -> (w3292:dbl)
    n2206 = local read "Trap AI FIFO Depth"() -> (w3416:u32)
    n2207 = local read "Number of APDs"() -> (w3092:u8)
    n2208 = Decimate 1D Array(w3189) -> (w3186:u16[], w3188:u16[], w3187:u16[])
    n2209 = feedback #3(0.0) -> (w3218:dbl)
    n2210 = Add(x=w3292, y=w3218) -> (x+y=w3390:dbl)
    n2211 = feedback-in #3(w3390) -> ()
    n2212 = To Time Stamp(1:w3218) -> (0:w3217:timestamp)
    n2213 = Subtract(x=w3416, y=w3291) -> (x-y=w3415:u32)
    n2214 = To Unsigned Long Integer(number=w3186) -> (unsigned 32bit integer=w3185:u32[])
    n2215 = Join Numbers(hi=w3188, lo=w3187) -> ((hi.lo)=w3184:u32[])
    n2216 = Divide(x=w3414, y=w3415) -> (x/y=w3413:dbl)
    "Buffer Status" <- w3413
    n2217 = case "Deinterlace APD signals" shown="3, Default" w3092 {
      tunnel: [w3426 w3432] -> w3069
      tunnel: w3260 -> [w3427 w3431]
      tunnel: [w3425 w3430] -> w3068
      tunnel: [w3424 w3428] -> w3075
      frame 3, Default {
        n2218 = Decimate 1D Array "APD signals"(w3427) -> (w3426:u32[], w3425:u32[], w3424:u32[])
      }
      frame 2 {
        n2219 = Decimate 1D Array "APD signals"(w3431) -> (w3432:u32[], w3430:u32[])
        n2220 = Multiply(x=w3430, y=u32 0) -> (x*y=w3428:u32[])
      }
    }
    n2221 = Join Numbers(hi=w3185, lo=w3184) -> ((hi.lo)=w3178:u64[])
    n2222 = call "IR AOM word to freq - vec.vi"("Frequency Word In (double vec)"=w3178) -> ("Frequency Out"=w3224:dbl[])
    n2223 = Equal?(x=w3413, y=1.0) -> (x = y?=w3411:bool)
    n2224 = case "Alert buffer overflow" shown="True" w3411 {
      frame False {
      }
      frame True {
        n2225 = call <vilib>:"Beep.vi"() -> ()  [unwired: 3 in, 9 out]
        "Overflow (data lost)" <- TRUE ("Overflow (data lost)")
      }
    }
    n2226 = Decimate 1D Array(w3224) -> (w3223:dbl[], w3222:dbl[])
    n2227 = Build Array(w3223, w3222) -> (w3221:dbl[][])
    n2228 = Bundle(w3069, w3068, w3075) -> (w3073:cluster{u32[], u32[], u32[]})  [unwired: 1 in]
    n2229 = Build Array(w3069, w3068, w3075) -> (w3350:u32[][])
    n2230 = for {
      tunnel: w3069 -> [w3422] mode=indexing
      n2231 = call "Smart Buffer (DBL) 1.vi"("new element [write]"=w3422, "mode"=T21."write") -> ()  [unwired: 4 in, 6 out]
    }
    n2232 = local read "APD Integration Time (s)"() -> (w3085:dbl)
    n2233 = To Double Precision Float(number=w3350) -> (double precision float=w3351:dbl[][])
    n2234 = feedback #4 "APD3"(w3075) -> (w3091:u32[])
    n2235 = feedback #5 "APD2"(w3068) -> (w3247:u32[])
    n2236 = feedback #6 "APD1"(w3069) -> (w3349:u32[])
    n2237 = Build Array (concatenate)(w3247, w3068) -> (w3246:u32[])
    n2238 = Build Array (concatenate)(w3091, w3075) -> (w3090:u32[])
    n2239 = Build Array (concatenate)(w3349, w3069) -> (w3346:u32[])
    n2240 = for {
      tunnel: w3068 -> [w3421] mode=indexing
      n2241 = call "Smart Buffer (DBL) 2.vi"("new element [write]"=w3421, "mode"=T21."write") -> ()  [unwired: 4 in, 6 out]
    }
    n2242 = Array Size(array=w3346) -> (size(s)=w3343:i32)
    n2243 = Array Size(array=w3069) -> (size(s)=w3345:i32)
    n2244 = Multiply(x=w3345, y="APD Ave N") -> (x*y=w3344:dbl)
    n2245 = Greater?(x=w3343, y=w3344) -> (0:w3347:bool)
    n2246 = Bundle("APD 1", "APD 2", "APD 3") -> (w3383:cluster{string, string, string})  [unwired: 1 out]
    n2247 = local read "Trap Sets"() -> (w3290:u32)
    n2248 = case shown="True" w3347 {
      tunnel: w3346 -> [w3724 w3733]
      tunnel: [w3724 w3731] -> w3297
      tunnel: w3344 -> [_ w3726]
      tunnel: w3343 -> [_ w3732]
      tunnel: w3246 -> [w3723 w3730]
      tunnel: [w3723 w3729] -> w3244
      tunnel: w3090 -> [w3722 w3728]
      tunnel: [w3722 w3725] -> w3086
      frame False {
      }
      frame True {
        n2249 = Subtract(x=w3732, y=w3726) -> (x-y=w3727:dbl)
        n2250 = Array Subset "APD3"(array=w3728, index=w3727, length=w3726) -> (w3725:u32[])
        n2251 = Array Subset "APD2"(array=w3730, index=w3727, length=w3726) -> (w3729:u32[])
        n2252 = Array Subset "APD1"(array=w3733, index=w3727, length=w3726) -> (w3731:u32[])
      }
    }
    n2253 = feedback-in #4(w3086) -> ()
    n2254 = feedback-in #5(w3244) -> ()
    n2255 = feedback-in #6(w3297) -> ()
    n2256 = Cluster To Array(cluster=w3383) -> (array=w3380:string[])
    n2257 = for "APD" {
      tunnel: w3351 -> [w3980] mode=indexing
      tunnel: w3085 -> [w3987]
      tunnel: [w3983] -> w3248 mode=indexing
      tunnel: "APD Disp. Scale" -> [w3984]
      tunnel: w3380 -> [w3982] mode=indexing
      tunnel: "APD Disp. Downsample" -> [w3978]
      tunnel: [w3981] -> w3379
      workers-P: _ -> [_]
      tunnel: w3217 -> [w3977]
      n2258 = call "integrate 1D array interval - double.vi"("Ave N"=w3978, "Array In"=w3980) -> ("Array Out"=w3979:dbl[])  [unwired: 1 out]
      n2259 = Multiply(x=w3987, y=w3978) -> (x*y=w3981:dbl)
      n2260 = Divide(x=w3979, y=w3984) -> (x/y=w3985:dbl[])
      n2261 = Bundle By Name("t0"=w3977, "Y"=w3985, "dt"=w3981) -> (w3986:waveform(dbl))  [unwired: 1 out]
      n2262 = Set Waveform Attribute(5:w3982, 6:"NI_ChannelName" ("name"), 7:w3986) -> (3:w3983:waveform(dbl))  [unwired: 1 in, 2 out]
    }
    "APD Display Period (s)" <- w3379
    n2263 = Reciprocal(x=w3379) -> (1/x=→"APD Display Freq. (Hz)":dbl)
    n2264 = case "Deinterlace trap data, average down PSD" shown="2" w3290 {
      tunnel: w3190 -> [w4005 w4070]
      tunnel: [w4002 w4067] -> w3283
      tunnel: [w4005 w4069] -> w3181
      tunnel: "Detector Type" -> [w4004 w4065]
      tunnel: [w4003 w4068] -> w3282
      tunnel: [w4001 w4066] -> w3388
      frame 1, Default {
        n2265 = Divide(x=w4005, y=3276.7) -> (x/y=w4006:dbl[])
        n2266 = Decimate 1D Array(w4006) -> (w4015:dbl[], w4014:dbl[], w4013:dbl[], w4012:dbl[], w4011:dbl[], w4010:dbl[], w4009:dbl[], w4008:dbl[])
        n2267 = case shown="\"IR-QPD + PSD + FB-QPD position\"" w4004 {
          tunnel: w4015 -> [w4039 w4064]
          tunnel: w4014 -> [w4038 w4063]
          tunnel: w4013 -> [w4023 w4041]
          tunnel: w4012 -> [w4024 w4051]
          tunnel: w4011 -> [w4037 w4062]
          tunnel: w4010 -> [w4036 w4061]
          tunnel: w4009 -> [w4020 w4042]
          tunnel: w4008 -> [w4019 w4040]
          tunnel: [w4018 w4048] -> w4003
          tunnel: [w4017 w4047] -> w4002
          tunnel: [w4016 w4046] -> w4001
          frame "IR-QPD + PSD + FB-QPD", Default {
            w4016 = 0  # Channel pattern
            n2268 = Divide(x=w4039, y=w4024) -> (x/y=w4026:dbl[])
            n2269 = Divide(x=w4038, y=w4024) -> (x/y=w4025:dbl[])
            n2270 = Divide(x=w4037, y=w4020) -> (x/y=w4022:dbl[])
            n2271 = Divide(x=w4036, y=w4019) -> (x/y=w4021:dbl[])
            n2272 = Build Array(w4026, w4025, w4024, w4023, w4022, w4021, w4020, w4019) -> (w4017:dbl[][])
            n2273 = Bundle("T1 Y", "T1 X", "T1 Sum", "FB Sum", "PSD Y", "PSD X", "PSD Y Sum", "PSD X Sum") -> (w4035:T41)  [unwired: 1 out]
            n2274 = Cluster To Array(cluster=w4035) -> (array=w4018:string[])
          }
          frame "IR-QPD + PSD + FB-QPD position" {
            w4046 = 3  # Channel pattern
            n2275 = Negate(x=w4042) -> (-x=w4043:dbl[])
            n2276 = Divide(x=w4064, y=w4051) -> (x/y=w4053:dbl[])
            n2277 = Divide(x=w4063, y=w4051) -> (x/y=w4052:dbl[])
            n2278 = Divide(x=w4062, y=w4042) -> (x/y=w4050:dbl[])
            n2279 = Divide(x=w4061, y=w4043) -> (x/y=w4049:dbl[])
            n2280 = Build Array(w4053, w4052, w4051, w4040, w4041, w4050, w4049, w4042) -> (w4047:dbl[][])
            n2281 = Bundle("T1 Y", "T1 X", "T1 Sum", "FB X", "FB Sum", "PSD Y", "PSD X", "PSD Y Sum") -> (w4060:T41)  [unwired: 1 out]
            n2282 = Cluster To Array(cluster=w4060) -> (array=w4048:string[])
          }
        }
      }
      frame 2 {
        n2283 = case shown="\"IR-QPD + PSD + FB-QPD X position\"" w4065 {
          tunnel: w4070 -> [w4132 w4204 w4275]
          tunnel: [w4071 w4195 w4206] -> w4069
          tunnel: [w4098 w4186 w4253] -> w4068
          tunnel: [w4097 w4149 w4220] -> w4067
          tunnel: [w4091 w4184 w4251] -> w4066
          frame "IR-QPD + PSD + FB-QPD", Default {
            w4091 = 1  # Channel pattern
            # "time average x2 the 4th signal and the 4 psd signals (detection laser)"
            # "deinterlace 3 signals from qpd"
            n2284 = Decimate 1D Array(w4132) -> (w4131:i16[], w4130:i16[], w4096:i16[], w4129:i16[], w4119:i16[], w4117:i16[], w4116:i16[], w4114:i16[])
            n2285 = Decimate 1D Array(w4096) -> (w4095:i16[], w4094:i16[])
            n2286 = Decimate 1D Array(w4131) -> (w4128:i16[], w4100:i16[])
            n2287 = Decimate 1D Array(w4130) -> (w4127:i16[], w4125:i16[])
            n2288 = Decimate 1D Array(w4129) -> (w4126:i16[], w4124:i16[])
            n2289 = call "downsample 1D array - double.vi"("Ave N"=2.0, "Array In"=w4119) -> ("Array Out"=w4118:dbl[])  [unwired: 1 out]
            n2290 = call "downsample 1D array - double.vi"("Ave N"=2.0, "Array In"=w4117) -> ("Array Out"=w4099:dbl[])  [unwired: 1 out]
            n2291 = call "downsample 1D array - double.vi"("Ave N"=2.0, "Array In"=w4116) -> ("Array Out"=w4115:dbl[])  [unwired: 1 out]
            n2292 = call "downsample 1D array - double.vi"("Ave N"=2.0, "Array In"=w4114) -> ("Array Out"=w4113:dbl[])  [unwired: 1 out]
            n2293 = Interleave 1D Arrays(w4128, w4127, w4126, w4100, w4125, w4124, w4095, w4094, w4118, w4099, w4115, w4113) -> (w4112:dbl[])
            n2294 = Divide(x=w4112, y=3276.7) -> (x/y=w4111:dbl[])
            n2295 = Decimate 1D Array(w4111) -> (w4110:dbl[], w4109:dbl[], w4108:dbl[], w4107:dbl[], w4106:dbl[], w4105:dbl[], w4093:dbl[], w4092:dbl[], w4104:dbl[], w4103:dbl[], w4102:dbl[], w4101:dbl[])
            n2296 = Divide(x=w4110, y=w4108) -> (x/y=w4078:dbl[])
            n2297 = Divide(x=w4109, y=w4108) -> (x/y=w4077:dbl[])
            n2298 = Divide(x=w4107, y=w4105) -> (x/y=w4076:dbl[])
            n2299 = Divide(x=w4106, y=w4105) -> (x/y=w4075:dbl[])
